vi "SAPHIR_DisableCode.vi"(6 "Variant in":variant, 7 "Shift Pressed?":bool, 8 "error in (no error)":errorcluster, 10 "QD Combo Box Ref":refnum<vi>, 11 "QD Launch VI Ref":refnum<vi>) -> (0 "error out":errorcluster, 4 "Variant out":variant)   [LabVIEW 2017]
doc: "PLUGIN_DESCRIPTION: Disable the selected code.\nPLUGIN_DEFAULT_SHORTCUT: Y"
uses:
  <userlib>/_LAVACR/Scripting Tools/Scripting Tools.lvlib
panel:
  in  "Undo Name":string="DisableCode"
  # "More informations on : https://decibel.ni.com/content/groups/saphir-toolkit"
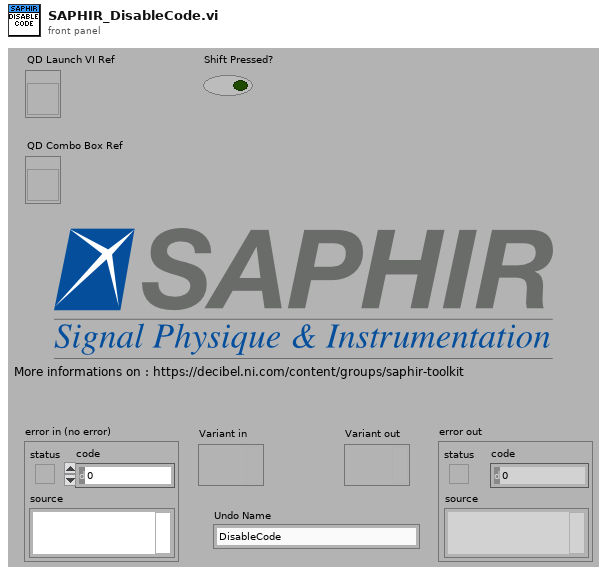
[diagram p1: front panel]
types:
  T1 = enum16{"Case Structure", "Stacked Sequence", "Event Structure", "Diagram Disable", "Conditional Disable", "While Loop", "For Loop", "Inplace Structure"}
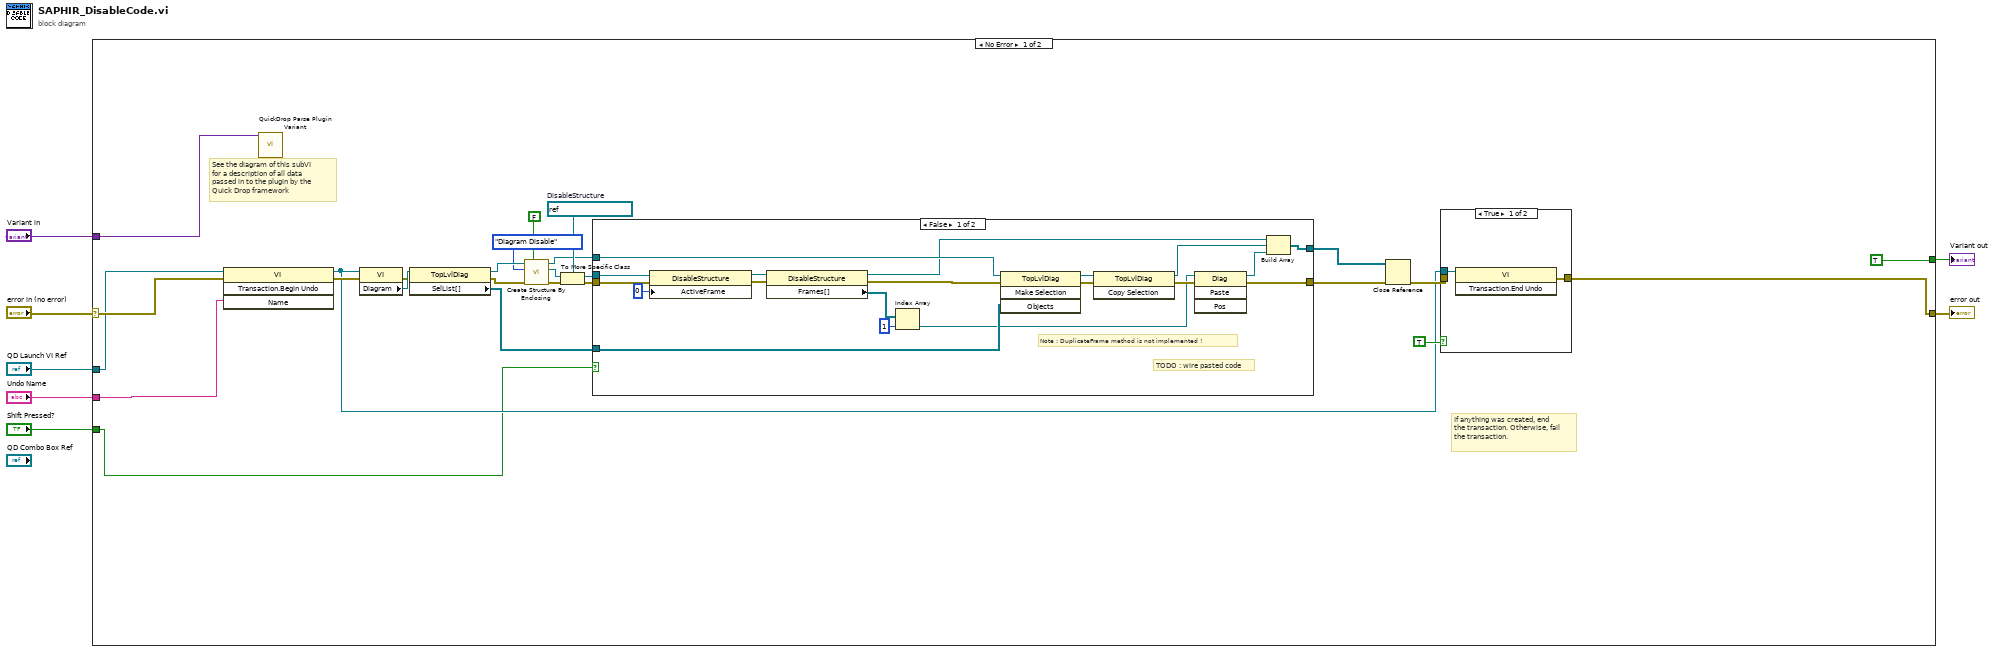
[diagram p0: block diagram]
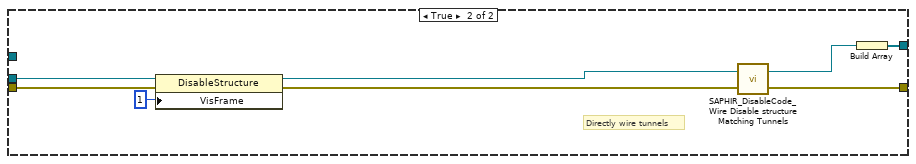
[diagram p2: hidden frame]
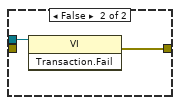
[diagram p3: hidden frame]
diagram:
  n1 = case shown="No Error" "error in (no error)" {
    selector: "error in (no error)" -> [w12 w65]
    tunnel: [w8 w65] -> w6
    tunnel: "QD Launch VI Ref" -> [w11 _]
    tunnel: "Variant in" -> [w13 _]
    tunnel: "Undo Name" -> [w10 _]
    tunnel: [TRUE _] -> w2
    tunnel: "Shift Pressed?" -> [w9 _]
    frame No Error {
      w19 = refnum<vi> refnum  # DisableStructure
      # "If anything was created, end the transaction. Otherwise, fail the transaction."
      # "See the diagram of this subVI for a description of all data passed in to the plugin by the Quick Drop framework"
      n2 = invoke class="VI" method="Transaction.Begin Undo"(reference=w11, error in=w12, "Name"=w10) -> (reference out=w28:refnum<vi>, error out=w32:errorcluster)  [unwired: 1 in, 2 out]
      n3 = call <vilib>:"QuickDrop Parse Plugin Variant.vi"("QDKS Variant in"=w13) -> ()  [unwired: 12 in, 3 out]
      n4 = property class="VI"(reference=w28, error in=w32) -> (error out=w25:errorcluster, "Diagram"=w26:refnum<vi>)  [unwired: 1 out]
      n5 = property class="TopLvlDiag"(reference=w26, error in=w25) -> (reference out=w27:refnum<vi>, error out=w31:errorcluster, "SelList[]"=w24:refnum<vi>[])
      n6 = call <userlib>:"Create Structure By Enclosing.vi"("Select everything except terminals ?"=FALSE, "error in (no error)"=w31, "Structure Type"=T1."Diagram Disable", "Diagram In"=w27) -> ("error out"=w20:errorcluster, "Structure Out"=w21:refnum<vi>, "Diagram Out"=w18:refnum<vi>)  [unwired: 5 in]
      n7 = To More Specific Class(target class=w19, reference=w21, error in=w20) -> (specific class reference=w16:refnum<vi>, error out=w15:errorcluster)
      n8 = case shown="False" w9 {
        tunnel: w24 -> [w52 _]
        tunnel: w18 -> [w51 _]
        tunnel: [w50 w58] -> w17
        tunnel: [w49 w60] -> w14
        tunnel: w16 -> [w37 w57]
        tunnel: w15 -> [w38 w56]
        frame False {
          # "Note : DuplicateFrame method is not implemented !"
          # "TODO : wire pasted code"
          n9 = property class="DisableStructure"(reference=w37, error in=w38, "ActiveFrame"=i16 0 ("Active Frame")) -> (reference out=w42:refnum<vi>, error out=w43:errorcluster)
          n10 = property class="DisableStructure"(reference=w42, error in=w43) -> (reference out=w34:refnum<vi>, error out=w36:errorcluster, "Frames[]"=w40:refnum<vi>[])
          n11 = Index Array(array=w40, index=u32 1 ("Visible Frame")) -> (element=w35:refnum<vi>)
          n12 = invoke class="TopLvlDiag" method="Make Selection"(reference=w51, error in=w36, "Objects"=w52) -> (reference out=w47:refnum<vi>, error out=w48:errorcluster)  [unwired: 1 in, 2 out]
          n13 = invoke class="TopLvlDiag" method="Copy Selection"(reference=w47, error in=w48) -> (reference out=w45:refnum<vi>, error out=w46:errorcluster)  [unwired: 1 in, 1 out]
          n14 = invoke class="Diag" method="Paste"(reference=w35, error in=w46) -> (reference out=w44:refnum<vi>, error out=w50:errorcluster)  [unwired: 2 in, 2 out]
          n15 = Build Array(w34, w45, w44) -> (w49:refnum<vi>[])
        }
        frame True {
          # "Directly wire tunnels"
          n16 = property class="DisableStructure"(reference=w57, error in=w56, "VisFrame"=u32 1 ("Visible Frame")) -> (reference out=w54:refnum<vi>, error out=w55:errorcluster)
          n17 = call <resource>:"SAPHIR_DisableCode_Wire Disable structure Matching Tunnels.vi"("Error In"=w55, "Frame Struct Refnum"=w54) -> ("error out"=w58:errorcluster, "Frame Struct Refnum"=w59:refnum<vi>)
          n18 = Build Array(w59) -> (w60:refnum<vi>[])
        }
      }
      n19 = Close Reference(reference=w14, error in (no error)=w17) -> (error out=w30:errorcluster)
      n20 = case shown="True" TRUE ("x") {
        tunnel: w28 -> [w61 w63]
        tunnel: [w62 w64] -> w8
        tunnel: w30 -> [_ _]
        frame True {
          n21 = invoke class="VI" method="Transaction.End Undo"(reference=w61) -> (error out=w62:errorcluster)  [unwired: 2 in, 2 out]
        }
        frame False {
          n22 = invoke class="VI" method="Transaction.Fail"(reference=w63) -> (error out=w64:errorcluster)  [unwired: 2 in, 2 out]
        }
      }
    }
    frame Error {
    }
  }
  "error out" <- w6
  "Variant out" <- w2
